vi "process-scan-data.vi"(8 "error in":errorcluster, 9 "output-data-path":path, 10 "scan_meta":T2, 11 "queue in":refnum<queue>) -> (0 "error out":errorcluster)   [LabVIEW 2017]
uses:
  controls/scan-mode-CTL.ctl
  controls/scan_input_meta_data.ctl
  controls/plot-channel-select.ctl
  controls/scan-plots.ctl
  controls/scan-plots-timeseries.ctl
  controls/time-series-graph-ref.ctl
panel:
  in  "plots":enum32{"Page 1", "Page 2"}(tab)
  out "channel-select":cluster{"W":dbl[], "Magnitude":dbl[]}[](graph) caption="Magnitude Graph"
  out "pixel-xsec-graph":cluster{"W":dbl[], "Magnitude":dbl[]}[](graph) caption="Magnitude Graph"
  out "Intensity Graph":dbl[][](graph)
  in  "Select-channel":T1=2 items=["x(k)", "y(k)", "deflection", "u_z"]
  out "x-axis":cluster{"W":dbl[], "Magnitude":dbl[]}[](graph) caption="Magnitude Graph"
  out "y-axis":cluster{"W":dbl[], "Magnitude":dbl[]}[](graph) caption="Magnitude Graph"
  out "z-deflection":cluster{"W":dbl[], "Magnitude":dbl[]}[](graph) caption="Magnitude Graph"
  out "z-control":cluster{"W":dbl[], "Magnitude":dbl[]}[](graph) caption="Magnitude Graph"
  in  "chunk-size":i32=400000
  in  "scan-mode":T3
  in  "detrend":bool=TRUE
  out "CURRENT-ROW":i32
  out "pixel-xsec-graph-ref":refnum<vi>
  out "IntensityGraph":refnum<vi>
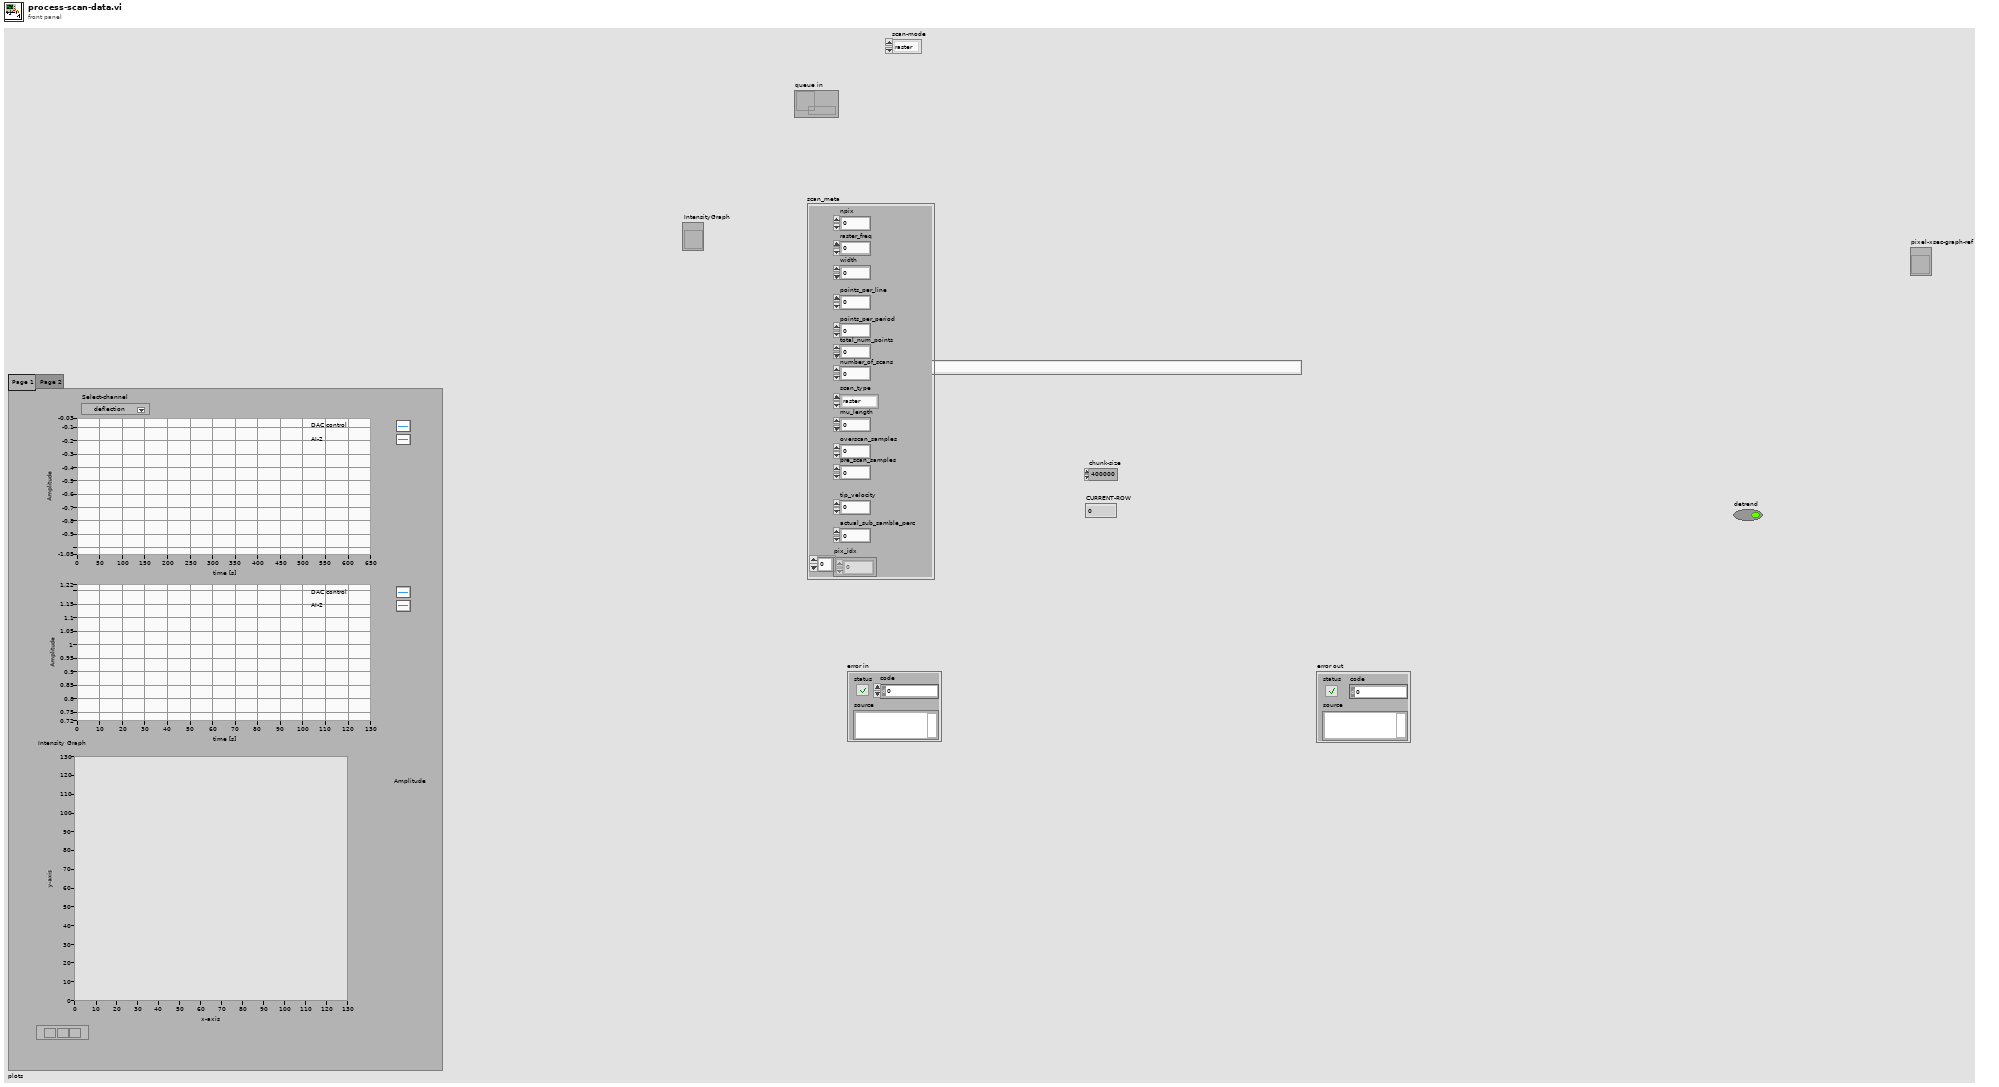
[diagram p1: front panel]
types:
  T1 = typedef "plot-channel-select.ctl" = u16
  T2 = typedef "scan_input_meta_data.ctl" = cluster{"npix":i64, "raster_freq":dbl, "width":dbl, "points_per_line":i64, "points_per_period":i64, "total_num_points":i64, "scan_type":T3, "number_of_scans":i64, "actual_sub_samble_perc":dbl, "mu_length":dbl, "tip_velocity":dbl, "pix_idx":i32[], "overscan_samples":i16, "pre_scan_samples":i16}
  T3 = typedef "scan-mode-CTL.ctl" = enum16{"raster", "CS"}
  T4 = typedef "scan-plots.ctl" = cluster{"IntensityGraph":refnum<vi>, "pixel-xsec-graph-ref":refnum<vi>, "time-series-plots":T5, "channel-select":refnum<vi>}
  T5 = typedef "scan-plots-timeseries.ctl" = cluster{"x-axis":T6, "y-axis":T6, "z-error":T6, "z-control":T6}
  T6 = typedef "time-series-graph-ref.ctl" = refnum<vi>
  T7 = enum16{"open", "replace", "create", "open or create", "replace or create", "replace or create with confirmation"}
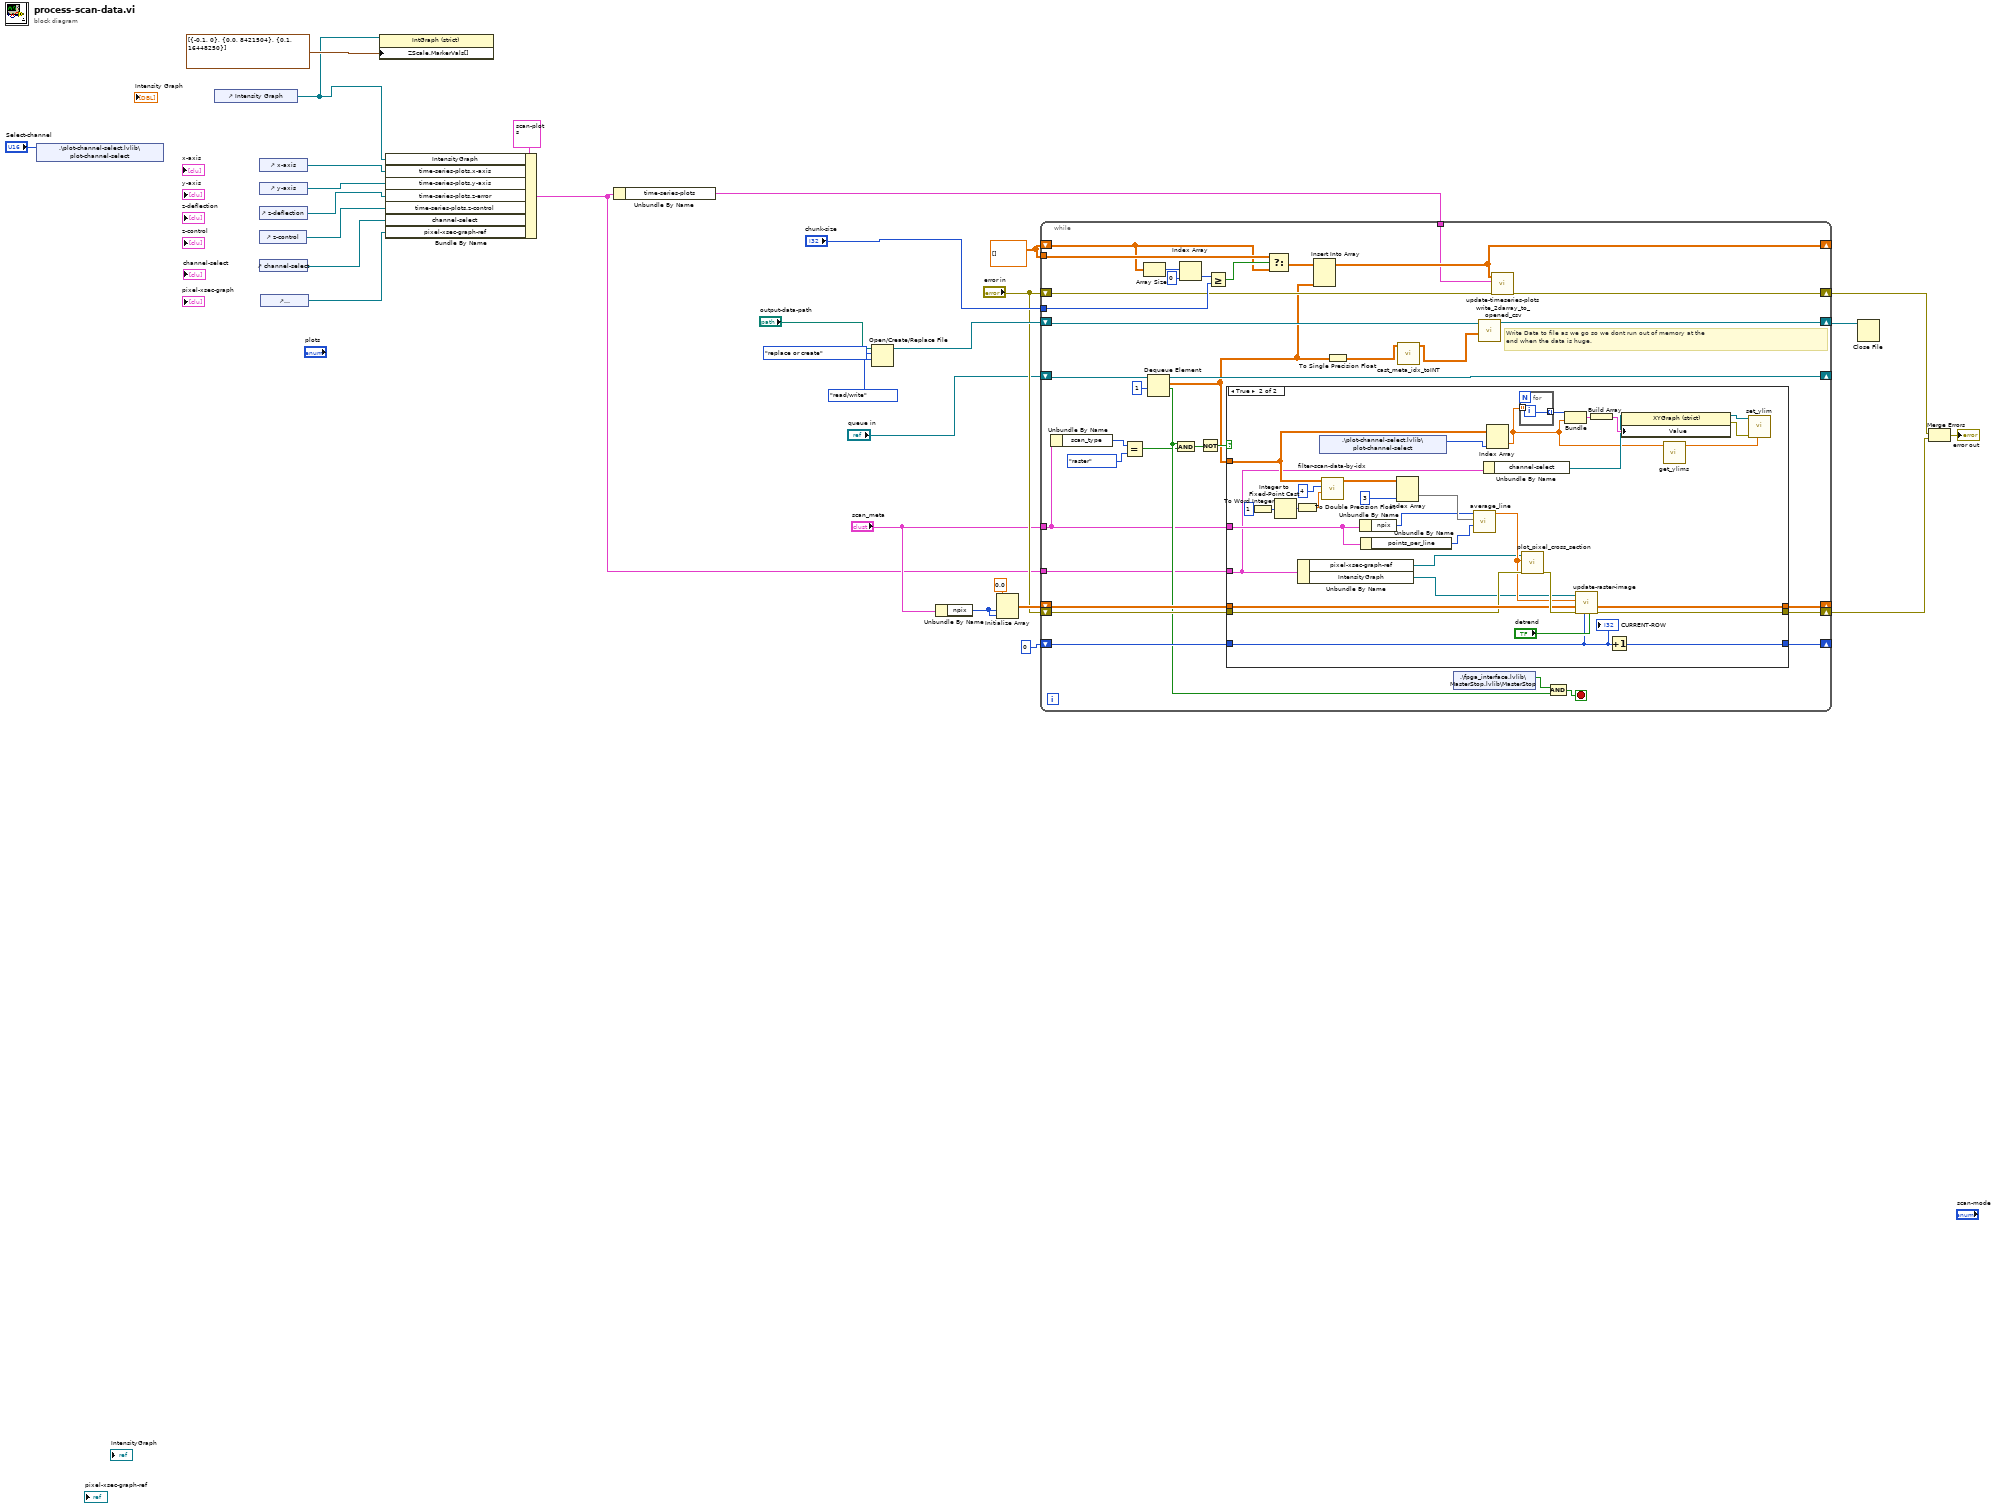
[diagram p0: block diagram]
diagram:
  w25 = dbl[][] [] ("old-data-out")
  n1 = shared-variable ".\\plot-channel-select.lvlib\\plot-channel-select"("Select-channel") -> ()  [unwired: 1 in, 1 out]
  n2 = control-ref of="Intensity Graph"() -> (w12:refnum<vi>)
  n3 = control-ref of="z-control"() -> (w8:refnum<vi>)
  n4 = control-ref of="x-axis"() -> (w11:refnum<vi>)
  n5 = control-ref of="y-axis"() -> (w10:refnum<vi>)
  n6 = control-ref of="z-deflection"() -> (w9:refnum<vi>)
  n7 = control-ref of="channel-select"() -> (w7:refnum<vi>)
  n8 = control-ref of="pixel-xsec-graph"() -> (w6:refnum<vi>)
  n9 = property on="Property Node" class="IntGraph (strict)"(reference=w12, "ZScale.MarkerVals[]"=cluster{dbl, u32}[] [{-0.1, 0}, {0.0, 8421504}, {0.1, 16448250}] ("Z Scale.Marker Values[]")) -> ()  [unwired: 1 in, 2 out]
  n10 = Bundle By Name(cluster=T4 {"IntensityGraph"=refnum, "pixel-xsec-graph-ref"=refnum, "time-series-plots"={"x-axis"=refnum, "y-axis"=refnum, "z-error"=refnum, "z-control"=refnum}, "channel-select"=refnum}, "IntensityGraph"=w12, "time-series-plots.x-axis"=w11, "time-series-plots.y-axis"=w10, "time-series-plots.z-error"=w9, "time-series-plots.z-control"=w8, "channel-select"=w7, "pixel-xsec-graph-ref"=w6) -> (w5:T4)
  n11 = Unbundle By Name(w5) -> ("time-series-plots"=w15:T5)
  n12 = Open/Create/Replace File(file path (use dialog)="output-data-path", operation (0:open)=T7."replace or create", access (0:read/write)=enum16{"read/write", "read-only", "write-only"}."read/write") -> (refnum out=w27:refnum<file>)  [unwired: 3 in, 2 out]
  n13 = Unbundle By Name("scan_meta") -> ("npix"=w18:i64)
  n14 = Initialize Array(0.0 ("element"), w18, w18) -> (w21:dbl[][])
  n15 = while {
    shift-right: [w63] -> _
    shift-left: "queue in" -> [w64]
    shift-right: [w62] -> w3
    shift-left: w27 -> [w34]
    shift-right: [w61] -> _
    shift-left: w21 -> [w60]
    shift-right: [w59] -> w2
    shift-left: "error in" -> [w58]
    shift-right: [w57] -> _
    shift-left: 0 ("disabled index (col)") -> [w56]
    shift-right: [w41] -> _
    shift-left: w25 -> [w50]
    tunnel: w25 -> [w51]
    tunnel: "chunk-size" -> [w42]
    tunnel: w15 -> [w40]
    shift-right: [w39] -> w1
    shift-left: "error in" -> [w38]
    tunnel: "scan_meta" -> [w37]
    tunnel: w5 -> [w36]
    stop <- w49 stop-if-true
    # "Write Data to file as we go so we dont run out of memory at the \nend when the data is huge."
    n16 = Unbundle By Name(w37) -> ("scan_type"=w30:T3)
    n17 = Equal?(x=w30, y=scan-mode-CTL."raster" ("scan-mode 2")) -> (x = y?=w44:bool)
    n18 = Array Size(array=w50) -> (size(s)=w55:i32[])
    n19 = Dequeue Element(queue=w64, timeout in ms (-1)=1) -> (queue out=w63:refnum<queue>, element=w33:dbl[][], timed out?=w45:bool)  [unwired: 1 in, 1 out]
    n20 = And(x=w45, y=w44) -> (x .and. y?=w46:bool)
    n21 = Index Array(array=w55, index=0) -> (element=w53:i32)
    n22 = Not(x=w46) -> (.not. x?=w47:bool)
    n23 = Greater Or Equal?(x=w53, y=w42) -> (x >= y?=w52:bool)
    n24 = case shown="True" w47 {
      tunnel: w33 -> [_ w92]
      tunnel: [w68 w100] -> w61
      tunnel: w60 -> [w68 w99]
      tunnel: [w67 w98] -> w59
      tunnel: w58 -> [w67 w97]
      tunnel: [w66 w95] -> w57
      tunnel: w56 -> [w66 w94]
      tunnel: w37 -> [_ w83]
      tunnel: w36 -> [_ w74]
      frame False {
      }
      frame True {
        n25 = To Word Integer(number=i16 1) -> (16bit integer=w86:i16)
        n26 = Integer to Fixed-Point Cast(integer=w86) -> (fixed-point=w85:fxp<+/-,16,5>)  [unwired: 1 in]
        n27 = To Double Precision Float(number=w85) -> (double precision float=w84:dbl)
        n28 = Unbundle By Name(w74) -> ("pixel-xsec-graph-ref"=w79:refnum<vi>, "IntensityGraph"=w78:refnum<vi>)
        n29 = shared-variable ".\\plot-channel-select.lvlib\\plot-channel-select"() -> (w80:T1)  [unwired: 1 in, 1 out]
        n30 = call "filter-scan-data-by-idx.vi"("scan-idx-as-double"=w84, "meta-column-idx"=4 ("disabled index (col)"), "data-in"=w92) -> ("filtered-data"=w90:dbl[][])  [unwired: 8 in]
        n31 = Unbundle By Name(w83) -> ("npix"=w82:i64)
        n32 = Unbundle By Name(w83) -> ("points_per_line"=w81:i64)
        n33 = Index Array(array=w90, index (col)=3 ("disabled index (col)")) -> (element=w88:dbl[])  [unwired: 1 in]
        n34 = call "average_line.vi"("data-pts-per-line"=w81, "raw-data-row"=w88, "number-of-pixels"=w82) -> ("avg-data-row"=w93:dbl[])  [unwired: 8 in]
        n35 = Unbundle By Name(w74) -> ("channel-select"=w73:refnum<vi>)
        n36 = Index Array(array=w92, index (col)=w80) -> (element=w70:dbl[])  [unwired: 1 in]
        n37 = for {
          tunnel: [w102] -> w77 mode=indexing
          tunnel: w70 -> [_] mode=indexing
          i -> [w102]
        }
        n38 = call "plot_pixel_cross_section.vi"("error in (no error)"=w97, "avg-data-row"=w93, "XYGraph"=w79) -> ("error out"=w101:errorcluster)  [unwired: 7 in, 1 out]
        n39 = Bundle(w77, w70) -> (w76:cluster{i32[], dbl[]})  [unwired: 1 in]
        n40 = call "update-raster-image.vi"("detrend"="detrend", "current-line"=w94, "error in (no error)"=w101, "Master-image-in"=w99, "avg-data-row"=w93, "IntensityGraph in"=w78) -> ("error out"=w98:errorcluster, "master-image-data-out"=w100:dbl[][])  [unwired: 3 in, 1 out]
        n41 = Build Array(w76) -> (w75:cluster{i32[], dbl[]}[])
        n42 = Increment(x=w94) -> (x+1=w95:i32)
        n43 = property on="Property Node" class="XYGraph (strict)"(reference=w73, "Value"=w75) -> (reference out=w72:refnum<vi>, error out=w71:errorcluster)  [unwired: 1 in]
        n44 = call "get_ylims.vi"("amplitudes"=w70) -> ("ylims"=w69:dbl[])  [unwired: 10 in]
        n45 = call "set_ylim.vi"("ylim"=w69, "error in"=w71, "figure (in)"=w72) -> ()  [unwired: 7 in, 2 out]
        "CURRENT-ROW" <- w94
      }
    }
    n46 = Select(t=w51, s=w52, f=w50) -> (s? t:f=w43:dbl[][])
    n47 = Insert Into Array(array=w43, new element=w33) -> (w41:dbl[][])  [unwired: 2 in]
    n48 = To Single Precision Float(number=w33) -> (single precision float=w32:sgl[][])
    n49 = call "cast_meta_idx_toINT.vi"("2D Data Out"=w32) -> ("output array"=w35:sgl[][])  [unwired: 10 in]
    n50 = shared-variable ".\\fpga_interface.lvlib\\MasterStop.lvlib\\MasterStop"() -> (w48:bool)  [unwired: 1 in, 1 out]
    n51 = call "write_2darray_to_opened_csv.vi"("Data_in"=w35, "file_ref_in"=w34) -> ("file_ref_out"=w62:refnum<file>)  [unwired: 9 in]
    n52 = call "update-timeseries-plots.vi"("error in (no error)"=w38, "input cluster"=w40, "data-in"=w41) -> ("error out"=w39:errorcluster)  [unwired: 8 in]
    n53 = And(x=w48, y=w45) -> (x .and. y?=w49:bool)
  }
  n54 = Close File(refnum=w3) -> ()  [unwired: 1 in, 2 out]
  n55 = Merge Errors(w1, w2) -> (→"error out":errorcluster)
